vi "OE1022D_Data Index.vi"(1 "Parameter Type":u16(ring) items=["A_X", "A_Y", "A_R", "A_θ", "A_Noise", "A_Freq", "A_XD1", "A_YD1", "A_RD1", "A_θD1", "A_XD2", "A_YD2", "A_RD2", "A_θD2", "B_X", "B_Y", "B_R", "B_θ", "B_Noise", "B_Freq", "B_XD1", "B_YD1", "B_RD1", "B_θD1", "B_XD2", "B_YD2", "B_RD2", "B_θD3", "ADC1", "ADC2", "ADC3", "ADC4"], 2 "Input Date Array":dbl[](array[numeric])) -> (0 "Parameter":dbl)   [LabVIEW 2019]
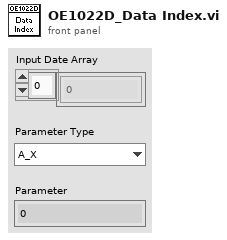
[diagram p1: front panel]
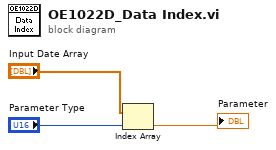
[diagram p0: block diagram]
diagram:
  n1 = Index Array(array="Input Date Array", index="Parameter Type") -> (element=→"Parameter":dbl)
